vi "collect_PH.vi"() -> (0 "Counts/s":i32, 1 "samples":i32, 2 "wrap":i32)   [LabVIEW 2013]
panel:
  out "dig here?":bool
  # "do i even need you </3"
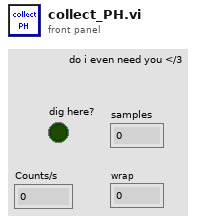
[diagram p1: front panel]
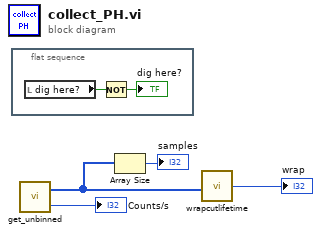
[diagram p0: block diagram]
diagram:
  n1 = flat-sequence {
    frame #0 {
      n2 = local read "dig here?"() -> (w5:bool)
      n3 = Not(x=w5) -> (.not. x?=→"dig here?":bool)
    }
  }
  n4 = call "get_unbinned.vi"() -> ("Counts/s"=→"Counts/s":i32, "Data"=w2:u8[])
  n5 = Array Size(array=w2) -> (size(s)=→"samples":i32)
  n6 = call "wrapcutlifetime.vi"("raw data"=w2) -> ("wrap"=→"wrap":i32)
